vi "Test Broadcast Debug Log Not Filtered by Inacitve Is Receive.vi"(8 "error in (no error)":errorcluster, 11 "Test Case In":refnum<class "Debugger Test.lvclass">) -> (0 "error out":errorcluster, 3 "Test Case Out":refnum<class "Debugger Test.lvclass">)   [LabVIEW 2020, in "Debugger Test.lvclass"]
uses:
  Debugger Test.lvclass
  C:/Program Files (x86)/National Instruments/LabVIEW 2020/vi.lib/Astemes/LUnit/Test Case.lvclass
  source/Debugger/Debugger.lvclass
  C:/Users/anton/Documents/GitHub/triarc-debugger/source/Process/Debug Process.lvclass
  source/Debug Data/Raw Debug Data.ctl
  source/Debug Data/Debug Data.lvclass
  source/Debug Data/Debug Data.lvclass/Debug Data.ctl
  source/Process/Debug Process.lvclass/Debug Process.ctl
  <vilib>/Astemes/LUnit/Test Case.lvclass/Test Case.ctl
  <vilib>/Astemes/LUnit/LUnit Assertion Result.lvclass/LUnit Assertion Result.ctl
  <vilib>/Astemes/LUnit/LUnit Test Case Result.lvclass/LUnit Test Case Result.ctl
  <vilib>/Astemes/LUnit/LUnit Method Result.lvclass/LUnit Method Result.ctl
  01074fa8-ee8a-411d-bc8b-fc92c4f90959.vi
  source/Process/Public/Lifecycle/Get Lifecycle State.vi
  source/Process/Private/SubVIs/Wait for finish.vi
  source/Process/Protected/Messaging/Enqueue Message.vi
  source/Process/Private/SubVIs/Set Lifecycle State.vi
  <vilib>/Astemes/LUnit/Palette/Pass.vi
  <vilib>/Astemes/LUnit/Palette/Fail.vi
  <vilib>/Astemes/LUnit/Compare Variants.vi
  <vilib>/Astemes/LUnit/Describe Comparison.vi
  <vilib>/Astemes/LUnit/Set Assertion Type.vi
  <vilib>/Utility/error.llb/Clear Errors.vi
  <vilib>/Astemes/LUnit/Add test result.vi
  <vilib>/Astemes/LUnit/LUnit Write Passed.vi
  <vilib>/Astemes/LUnit/LUnit Write Message.vi
  <vilib>/Astemes/LUnit/LUnit Write Description.vi
  <vilib>/Astemes/LUnit/Variant to string.vi
  <vilib>/Astemes/LUnit/LUnit Write Assertion Type.vi
  <vilib>/Astemes/LUnit/LUnit Record Assertion Result.vi
  <vilib>/Astemes/LUnit/LUnit Aggregate Assertion Results.vi
  <vilib>/Astemes/LUnit/Assertion Result/LUnit Read Status.vi
  <vilib>/Astemes/LUnit/LUnit Read Message.vi
  <vilib>/Astemes/LUnit/LUnit Read Description.vi
  <vilib>/Astemes/LUnit/Method Result/LUnit Merge Status.vi
  <vilib>/Astemes/LUnit/LUnit Concatenate result strings.vi
  <vilib>/Utility/error.llb/Error Cluster From Error Code.vi
  <vilib>/Utility/Data Type/Get Type Information.vi
  <vilib>/Utility/LVClass/Get LV Class Name.vi
  <vilib>/Astemes/LUnit/LUnit Assertion Result.lvclass
  source/Process/Debug Process.lvclass
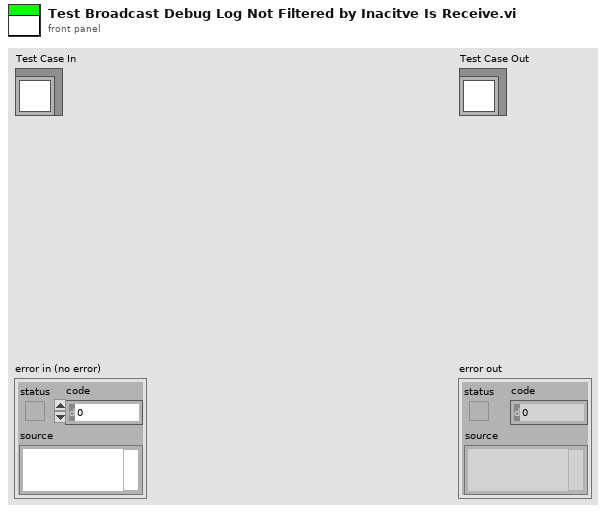
[diagram p1: front panel]
types:
  T1 = typedef "Debug Data.lvclass/Raw Debug Data.ctl" = cluster{"Action":string, "Call Chain":string, "Process":string, "Message":string, "Message Data":variant, "Time":dbl}
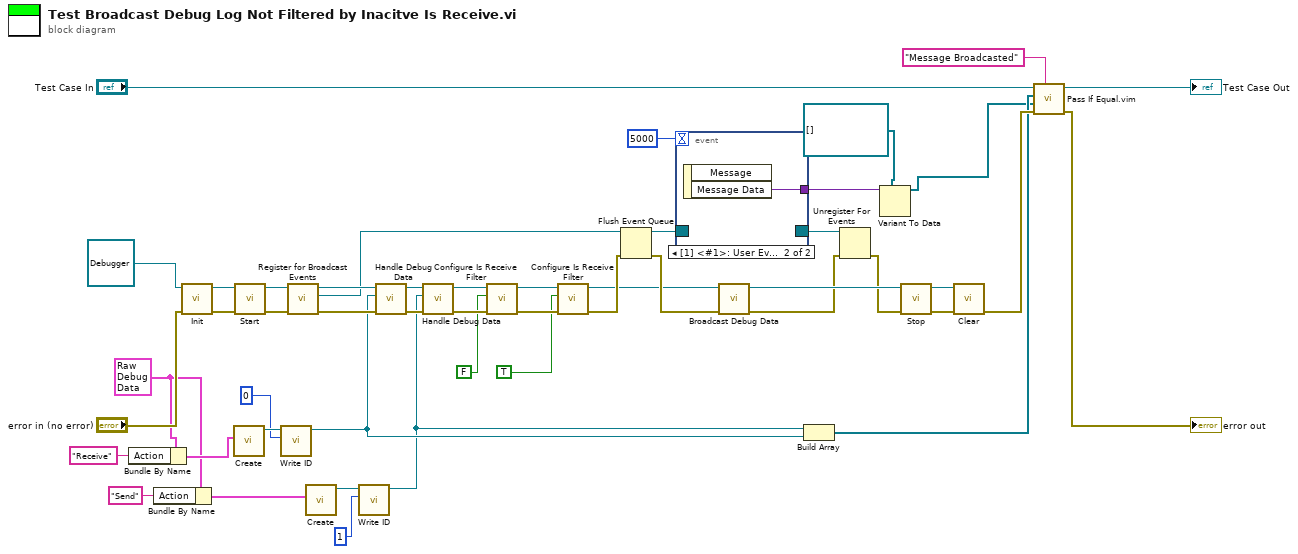
[diagram p0: block diagram]
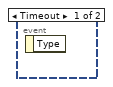
[diagram p2: hidden frame]
diagram:
  w17 = T1 {"Action"="", "Call Chain"="", "Process"="", "Message"="", "Message Data"=variant, "Time"=0.0} ("Debug Data Cluster")
  n1 = Bundle By Name(cluster=w17, "Action"="Receive" ("Process")) -> (w24:T1)
  n2 = Bundle By Name(cluster=w17, "Action"="Send" ("Process")) -> (w18:T1)
  n3 = call-dynamic "Init.vi"("error in (no error)"="error in (no error)", "Process In"=refnum<class "Debugger.lvclass"> refnum ("Debug Data Event In 2")) -> ("error out"=w44:errorcluster, "Process Out"=w45:refnum<class "Debugger.lvclass">)  [unwired: 8 in]
  n4 = call "Create.vi"("Debug Data Cluster"=w24) -> ("Debug Data out"=w30:refnum<class "Debug Data.lvclass">)  [unwired: 9 in, 1 out]
  n5 = call "Start.vi"("error in (no error)"=w44, "Process In"=w45) -> ("error out"=w42:errorcluster, "Process Out"=w43:refnum<class "Debugger.lvclass">)  [unwired: 7 in, 1 out]
  n6 = call "Write ID.vi"("ID"=u32 0, "Debug Data in"=w30) -> ("Debug Data out"=w4:refnum<class "Debug Data.lvclass">)  [unwired: 8 in, 1 out]
  n7 = call "Register for Broadcast Events.vi"("error in (no error)"=w42, "Process In"=w43) -> ("error out"=w41:errorcluster, "Event Registration Refnum Out"=w26:refnum<event-registration>, "Process Out"=w37:refnum<class "Debugger.lvclass">)  [unwired: 7 in]
  n8 = call "Create.vi"("Debug Data Cluster"=w18) -> ("Debug Data out"=w7:refnum<class "Debug Data.lvclass">)  [unwired: 9 in, 1 out]
  n9 = call "Write ID.vi"("ID"=u32 1, "Debug Data in"=w7) -> ("Debug Data out"=w3:refnum<class "Debug Data.lvclass">)  [unwired: 8 in, 1 out]
  n10 = call-dynamic "Handle Debug Data.vi"("error in (no error)"=w41, "Debug Data.lvclass"=w4, "Debug Data Event In"=w37) -> ("error out"=w21:errorcluster, "Debug Data Event Out"=w22:refnum<class "Debugger.lvclass">)  [unwired: 7 in]
  n11 = call-dynamic "Handle Debug Data.vi"("error in (no error)"=w21, "Debug Data.lvclass"=w3, "Debug Data Event In"=w22) -> ("error out"=w20:errorcluster, "Debug Data Event Out"=w15:refnum<class "Debugger.lvclass">)  [unwired: 7 in]
  n12 = call "Configure Is Receive Filter.vi"("error in (no error)"=w20, "Show Receive?"=FALSE ("Show Send?"), "Debugger In"=w15) -> ("error out"=w16:errorcluster, "Debugger Out"=w10:refnum<class "Debugger.lvclass">)  [unwired: 7 in]
  n13 = call "Configure Is Receive Filter.vi"("error in (no error)"=w16, "Show Receive?"=TRUE ("Show Send?"), "Debugger In"=w10) -> ("error out"=w11:errorcluster, "Debugger Out"=w9:refnum<class "Debugger.lvclass">)  [unwired: 7 in]
  n14 = Flush Event Queue(0:w26, 3:w11) -> (8:w25:refnum<event-registration>, 11:w27:errorcluster)  [unwired: 4 in, 1 out]
  n15 = event shown="[1] <#1>: User Event" {
    selector: w25 -> [_ _]
    dyn-events: [_ _] -> w32
    timeout: 5000 -> [_ _]
    tunnel: [_ w49] -> w29
    event Timeout {
      n16 = event-data() -> ()  [unwired: 1 in, 1 out]
    }
    event User Event {
      n17 = event-data() -> ("Message Data"=w49:variant)  [unwired: 1 in, 1 out]
    }
  }
  n18 = call "Broadcast Debug Data.vi"("error in (no error)"=w27, "Debugger in"=w9) -> ("error out"=w14:errorcluster, "Debugger out"=w40:refnum<class "Debugger.lvclass">)  [unwired: 8 in]
  n19 = Build Array(w3, w4) -> (w28:refnum<class "Debug Data.lvclass">[])
  n20 = Unregister For Events(event registration refnum=w32, error in=w14) -> (error out=w13:errorcluster)
  n21 = Variant To Data(type=refnum<class "Debug Data.lvclass">[] [] ("appended array"), Variant=w29) -> (data=w5:refnum<class "Debug Data.lvclass">[])  [unwired: 1 in, 1 out]
  n22 = call "Stop.vi"("error in (no error)"=w13, "Process In"=w40) -> ("error out"=w38:errorcluster, "Process Out"=w39:refnum<class "Debugger.lvclass">)  [unwired: 7 in, 1 out]
  n23 = call-dynamic "Clear.vi"("error in (no error)"=w38, "Process In"=w39) -> ("error out"=w34:errorcluster)  [unwired: 9 in]
  n24 = call "Pass If Equal.vim"("Description"="Message Broadcasted", "error in (no error)"=w34, "Actual"=w5, "Expected"=w28, "LUnit Test Case In"="Test Case In") -> ("error out"=→"error out":errorcluster, "LUnit Test Case Out"=→"Test Case Out":refnum<class "Debugger Test.lvclass">)  [unwired: 5 in]
